vi "Error Test Channel Number.vi"(7 "reset (F)":bool, 8 "error in":errorcluster, 10 "channel #":u16) -> (0 "error out":errorcluster)   [LabVIEW 2020, in "ARINC 429 Import.lvlib"]
uses:
  ARINC 429 Import.lvlib
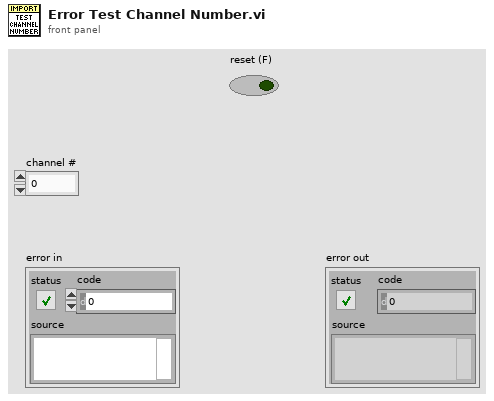
[diagram p1: front panel]
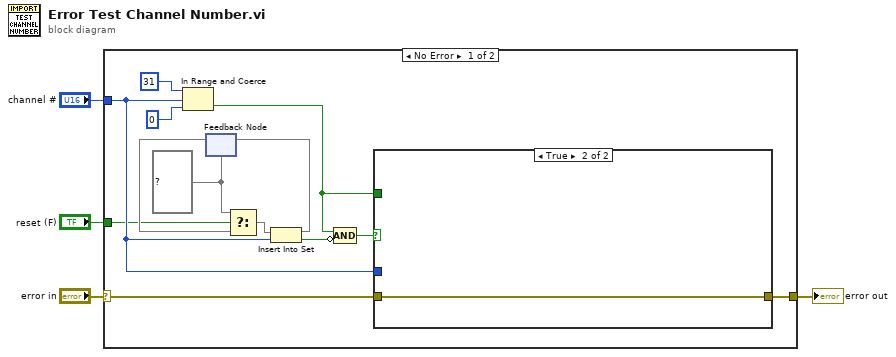
[diagram p0: block diagram]
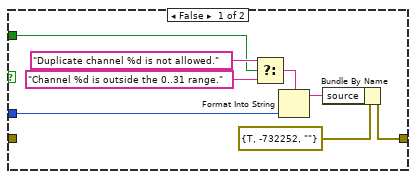
[diagram p2: hidden frame]
diagram:
  n1 = case shown="No Error" "error in" {
    selector: "error in" -> [w16 w27]
    tunnel: [w15 w27] -> w3
    tunnel: "channel #" -> [w17 _]
    tunnel: "reset (F)" -> [w5 _]
    frame No Error {
      w6 = set{u16} {} ("set in")
      n2 = In Range and Coerce(upper limit=u16 31 ("Channel #"), x=w17, lower limit=u16 0 ("Channel #")) -> (In Range?=w9:bool)  [unwired: 1 out]
      n3 = feedback #1(w6) -> (w8:set{u16})
      n4 = Select(t=w6, s=w5, f=w8) -> (s? t:f=w7:set{u16})
      n5 = Insert Into Set(10:w17, 11:w7) -> (2:w11:bool, 3:w12:set{u16})
      n6 = feedback-in #1(w12) -> ()
      n7 = Compound Arithmetic op=AND(w9, invert w11) -> (w10:bool)
      n8 = case shown="True" w10 {
        tunnel: w16 -> [_ w26]
        tunnel: [w18 w26] -> w15
        tunnel: w17 -> [w24 _]
        tunnel: w9 -> [w20 _]
        frame False {
          n9 = Select(t="Duplicate channel %d is not allowed." ("source"), s=w20, f="Channel %d is outside the 0..31 range." ("source")) -> (s? t:f=w19:string)
          n10 = Format Into String(format string=w19, w24) -> (resulting string=w25:string)  [unwired: 2 in, 1 out]
          n11 = Bundle By Name(cluster=errorcluster {"status"=TRUE, "code"=-732252, "source"=""} ("error constant"), "source"=w25) -> (w18:errorcluster)
        }
        frame True {
        }
      }
    }
    frame Error {
    }
  }
  "error out" <- w3
